vi "Measure_Synthetic_Jet_Select_Channel.vi"(3 "Mode":T1=enum."Run VI", 5 "Traverse line In":T3={"Start X"=0.0, "Start Y"=0.0, "Start Z"=0.0, "End X"=nan, "End Y"=nan, "End Z"=nan, "No. of pts."=5, "Spacing"=enum."Linear", "Filename"=path "C:/EnFlo_Data_Local/2013/Aero_Tunnel/Nick_Martin/Results/01-2013/QA_test_I.xls", "Tunnel Speed"=nan, "Averaging time (min)"=0.08, "Extra Commands"="", "Specific Arguments"="Measure_Synthetic_Jet.vi; 200; 1000; 100", "Emission Rate (l/min)"=nan, "Trace Gas Concentration (%)"=nan, "Density Ratio"="  ---------", "Comments"="", "Row No"=0, "Row Type Selector"=enum."Run VI Named:", "Completion time"="17:12  07-01-2013", "Row Duration (mins)"=4.483248000000001, "No. of Valid pts."=5, "Meas Setup File"="LDA_SJ_A.xls"} {"Row Duration (mins)" format="%#.1f"; "Row No" min=0; "Trace Gas Concentration (%)" min=0.0 format="%#.2f"; "Emission Rate (l/min)" format="%#.2f"; "Tunnel Speed" format="%#.2f"; "Start X" format="%#.2f"; "Start Y" format="%#.2f"; "Start Z" format="%#.2f"; "End X" format="%#.2f"; "End Y" format="%#.2f"; "End Z" format="%#.2f"; "Averaging time (min)" min=0.0 format="%#.2f"}) -> (0 "Error Message":string, 1 "Status":T2, 2 "Traverse line Out":T3={"Start X"=0.0, "Start Y"=0.0, "Start Z"=0.0, "End X"=nan, "End Y"=nan, "End Z"=nan, "No. of pts."=5, "Spacing"=enum."Linear", "Filename"=path "C:/EnFlo_Data_Local/2013/Aero_Tunnel/Nick_Martin/Results/01-2013/QA_test_I.xls", "Tunnel Speed"=nan, "Averaging time (min)"=0.08, "Extra Commands"="", "Specific Arguments"="Measure_Synthetic_Jet.vi; 200; 1000; 100", "Emission Rate (l/min)"=nan, "Trace Gas Concentration (%)"=nan, "Density Ratio"="  ---------", "Comments"="", "Row No"=0, "Row Type Selector"=enum."Run VI Named:", "Completion time"="17:12  07-01-2013", "Row Duration (mins)"=4.483248000000001, "No. of Valid pts."=5, "Meas Setup File"="LDA_SJ_A.xls"} {"Row Duration (mins)" format="%#.1f"; "Row No" min=0; "Trace Gas Concentration (%)" min=0.0 format="%#.2f"; "Emission Rate (l/min)" format="%#.2f"; "Tunnel Speed" format="%#.2f"; "Start X" format="%#.2f"; "Start Y" format="%#.2f"; "Start Z" format="%#.2f"; "End X" format="%#.2f"; "End Y" format="%#.2f"; "End Z" format="%#.2f"; "Averaging time (min)" min=0.0 format="%#.2f"})   [LabVIEW 2013]
uses:
  Gen Trav/Traverse_cluster.ctl
  Gen Trav/Spacing.ctl
  Controls/Multi_run_mode.ctl
  Gen Trav/Multi_Run_Status.ctl
  Controls/User_Specific_mode.ctl
  Controls/Setup.ctl
  Controls/Save_Data.ctl
  ADAM Client/Sub VIs/ADAM Controls/Update_scan_value.ctl
  <vilib>/Analysis/1siggen.llb/Ramp Pattern by Samples.vi
  Globals/Meas_global.vi
  Globals/Synthetic_jet_global.vi
  Globals/Extra_Commands_Global.vi
  <vilib>/Analysis/NI_AALBase.lvlib
panel:
  in  "Ch2 Phse average? (ON for AM on Ch2)":bool
  in  "Enter SJ Data?":bool
  in  "Stop Button":bool
  out "Last Meas Point":bool=TRUE
  out "Data":cluster{"Ramp Pattern":dbl[], dbl[]}[](graph)
  in  "Channels to Analyse":i32[](listbox)=[0, 2]
  in  "VISA resource name":refnum<visa-resource-name>="USB0::0x0699::0x0347::C036837::INSTR"
  out "First Meas Point":bool=TRUE
  # "Check the Multirun in order to populate these Channels!"
  # "X           Y            Z"
  # "Start"
  # "End"
  # "X           Y            Z"
  # "Start"
  # "End"
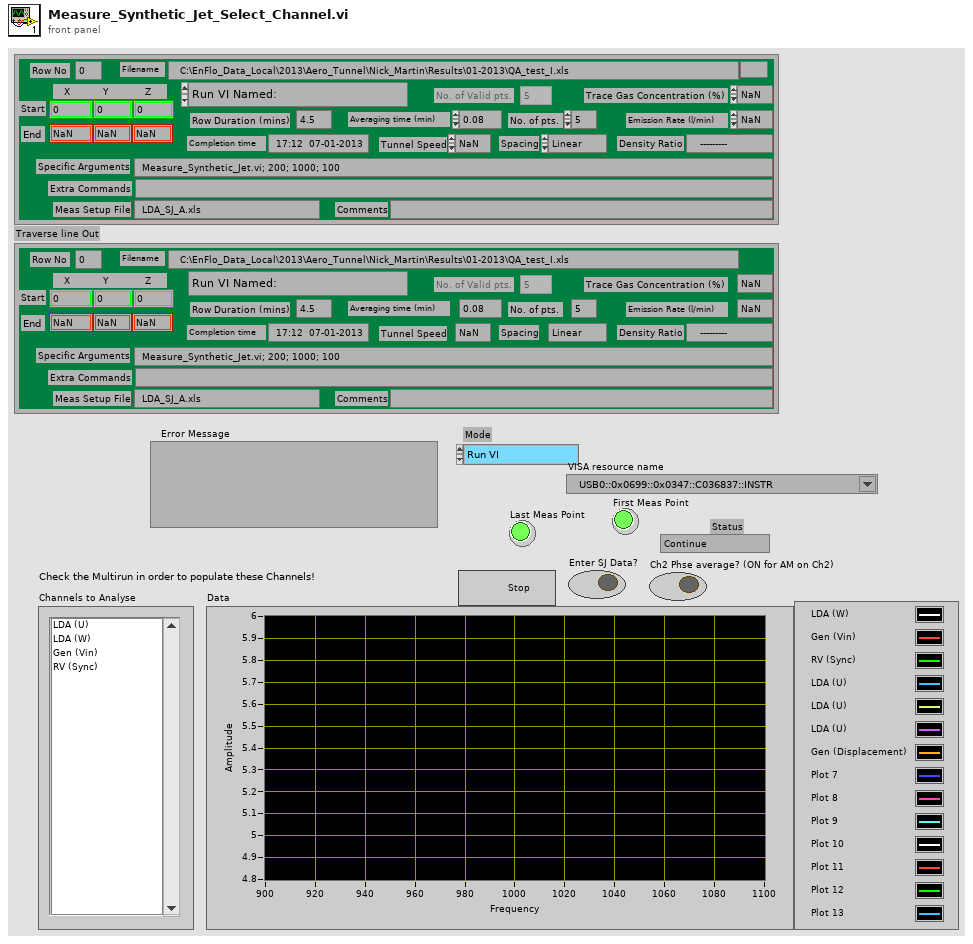
[diagram p1: front panel]
types:
  T1 = typedef "User_Specific_mode.ctl" = enum16{"Check VI only", "Run VI"}
  T2 = typedef "Multi_Run_Status.ctl" = enum16{"Continue", "Jump to Next Point", "Jump to Next Row", "Jump To Fall Back", "Terminate Run"}
  T3 = typedef "Traverse_cluster.ctl" = cluster{"Start X":dbl, "Start Y":dbl, "Start Z":dbl, "End X":dbl, "End Y":dbl, "End Z":dbl, "No. of pts.":i32, "Spacing":T4, "Filename":path, "Tunnel Speed":dbl, "Averaging time (min)":dbl, "Extra Commands":string, "Specific Arguments":string, "Emission Rate (l/min)":dbl, "Trace Gas Concentration (%)":dbl, "Density Ratio":string, "Comments":string, "Row No":i32, "Row Type Selector":T5, "Completion time":string, "Row Duration (mins)":dbl, "No. of Valid pts.":i32, "Meas Setup File":string}
  T4 = typedef "Spacing.ctl" = enum16{"Linear", "Log", "Gauss", "Specified", "N/A"}
  T5 = typedef "Multi_run_mode.ctl" = enum16{"Move Traverse Only", "Set Tunnel Speed Only", "Set Source Only", "Set Measurement Conditions", "Single Measurement", "Vertical Profile", "Lateral Profile", "Longitudinal Profile", "Explore Volume", "Multi-Axis Profile", "Auto Calibrate", "Meas Fast FID Bkgnd", "Check Beam Power", "Scanning Valve Measurement", "Run VI Named:", "Set ADAM Ch", "Wait (minutes)", "Send Message", "Synchronize With:", "Fall Back to this Row", "Turn Off Row Repeating", "Blank Row", "Traverse 3D Volume"}
  T6 = typedef "Analysis_info_cluster.ctl" = cluster{"Colour":u32, "Inst type":T7, "Inst name":string, "Symbol":string, "Code name":string, "Extra Info":string, "Inst Array":T8, "Extra Titles":string[], "Extra Values":string[], "U":dbl, "u^2":dbl, "u^3":dbl, "u^4":dbl, "Skew_u":dbl, "Kurt_u":dbl, "Sd Error in Mean":dbl, "% u'/U":dbl, "X":dbl, "Y":dbl, "Z":dbl, "Timescale integral to 25%":dbl, "Sd Error in Variance":dbl, "Calib File":path, "Calib Constants":dbl[], "Output Position":bool, "Full Stats":bool, "Av Sampling Rate":dbl, "Av No of Samples":dbl, "Total Meas Time (s)":dbl, "ADAM Ch Name":string}
  T7 = typedef "Inst_type.ctl" = enum16{"Propeller anemometer", "Raw voltage", "Pressure Transducer", "Pitot-static tube", "Preston tube", "Hot wire", "Cross wire 1", "Cross wire 2", "Generic Linear", "Generic Polynomial", "Generic BackPoly", "Fast FID", "Thermocouple", "Cold wire", "Pulsed Wire", "LDA Vel", "LDA Tran time", "LDA Arr time"}
  T8 = typedef "Instrument_Array.ctl" = enum16{"PWA", "LDA", "Analogue"}
  T9 = typedef "Save_Data.ctl" = enum16{"Save No Data", "Save Data"}
  T10 = typedef "Setup.ctl" = enum16{"Run Program", "Show Setup", "Save Current Setup", "Setup Front Panel"}
  T11 = typedef "SJ_Data_Cluster.ctl" = cluster{"Do (mm)":dbl, "Dc (mm)":dbl, "Ho (mm)":dbl, "Hc (mm)":dbl, "K":dbl, "beta":dbl, "Vc (m^3)":dbl, "Vo (m^3)":dbl}
  T12 = typedef "Update_scan_value.ctl" = cluster{"Channel Name":string, "New Value":dbl}
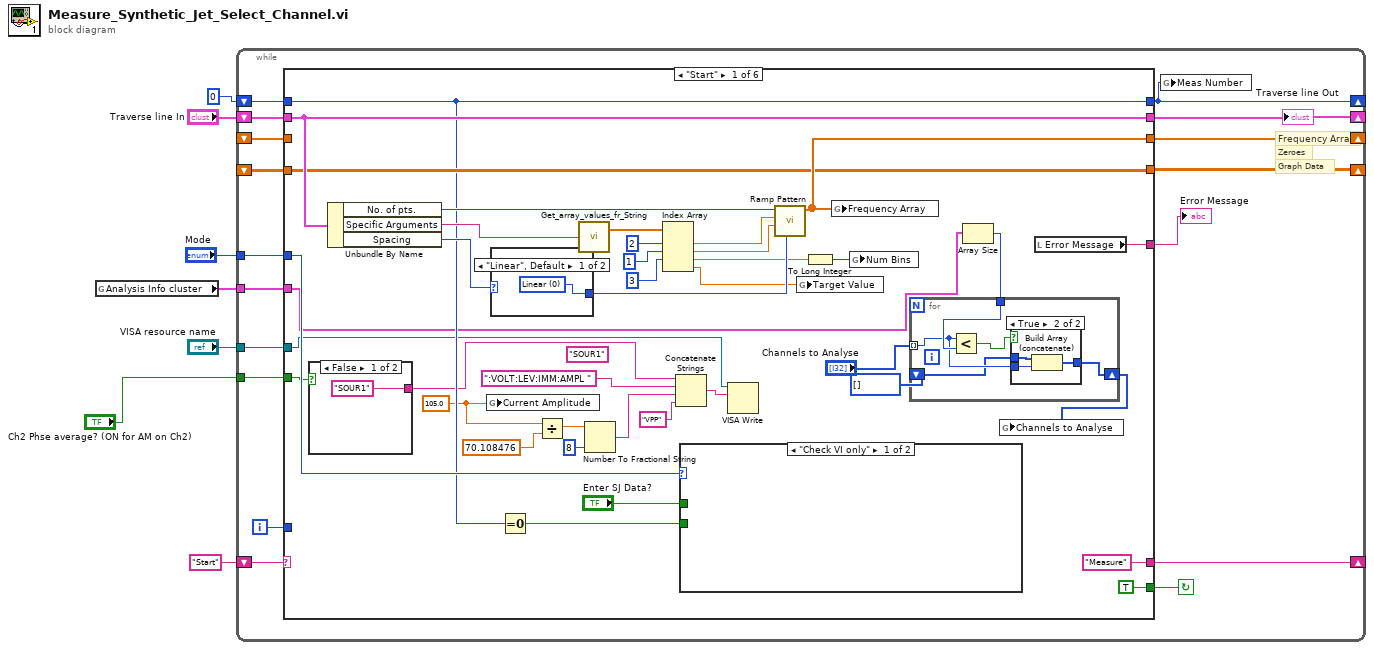
[diagram p0: block diagram]
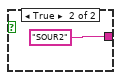
[diagram p2: hidden frame]
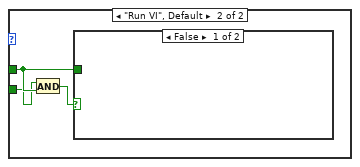
[diagram p4: hidden frame]
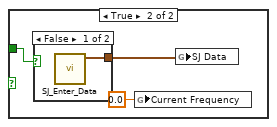
[diagram p5: hidden frame]
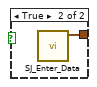
[diagram p6: hidden frame]
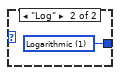
[diagram p7: hidden frame]
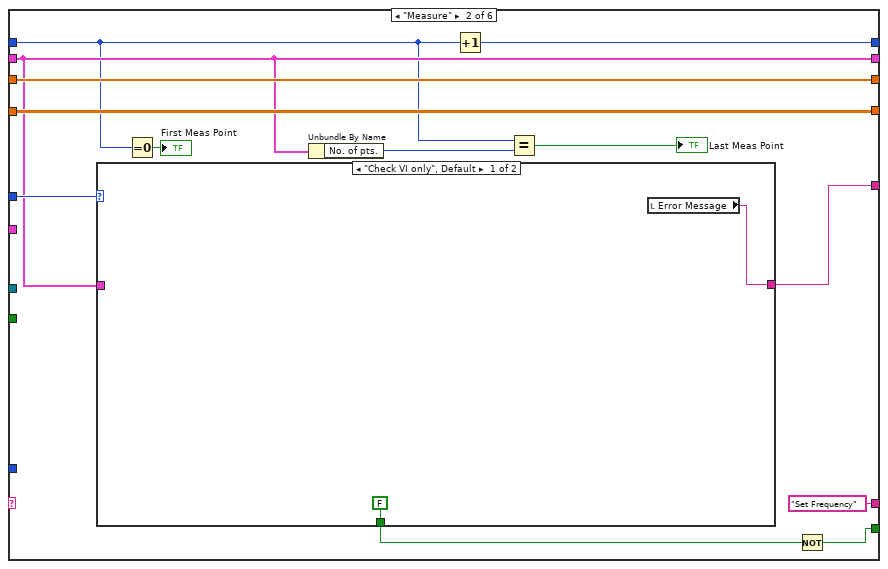
[diagram p8: hidden frame]
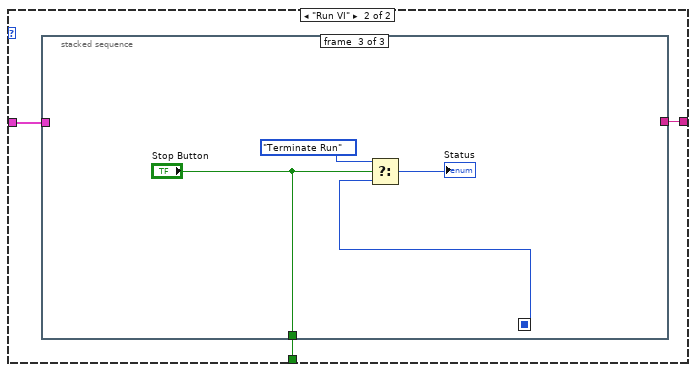
[diagram p9: hidden frame]
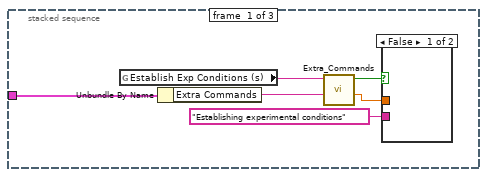
[diagram p10: hidden frame]
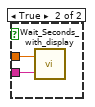
[diagram p11: hidden frame]
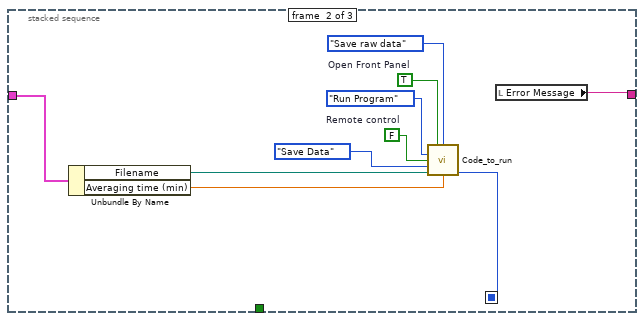
[diagram p12: hidden frame]
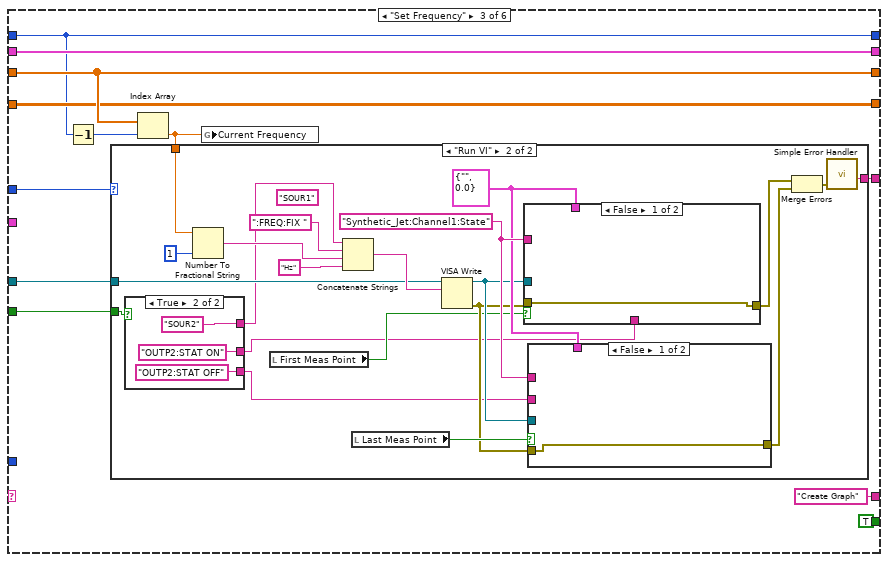
[diagram p13: hidden frame]
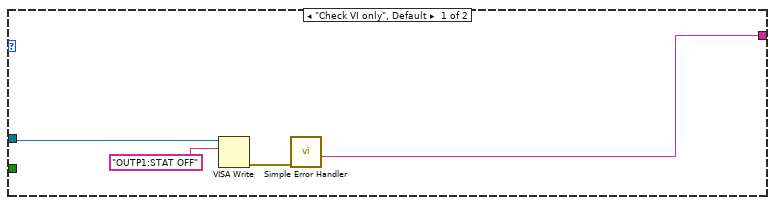
[diagram p14: hidden frame]
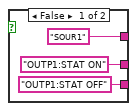
[diagram p15: hidden frame]
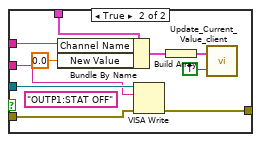
[diagram p16: hidden frame]
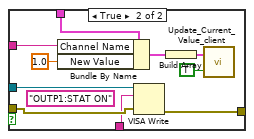
[diagram p17: hidden frame]
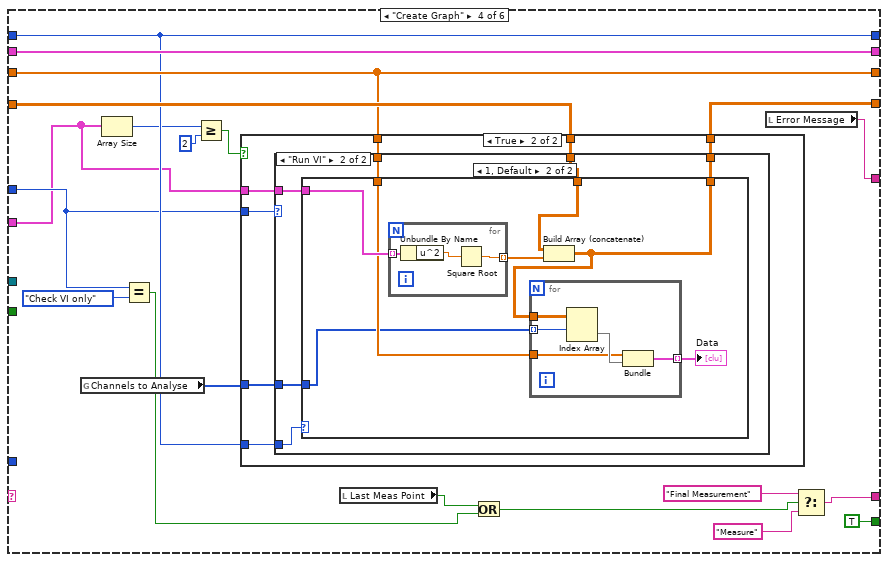
[diagram p18: hidden frame]
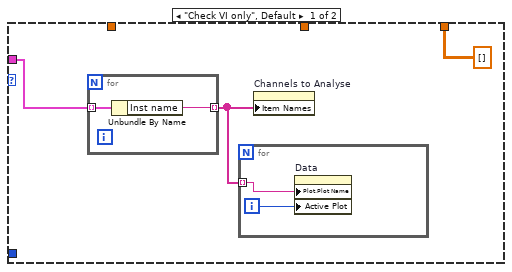
[diagram p20: hidden frame]
diagram:
  # "Graph Data"
  # "Zeroes"
  # "Frequency Array"
  n1 = global read "Meas_global.vi" "Analysis Info cluster"() -> (w2:T6[])
  n2 = while {
    shift-right: [w23] -> _
    shift-left: "Start" -> [w22]
    shift-right: [w21] -> w6
    shift-left: "Traverse line In" -> [w25]
    shift-right: [w20] -> _
    shift-left: _ -> [w19]
    tunnel: "Mode" -> [w18]
    tunnel: "VISA resource name" -> [w16]
    shift-right: [w15] -> _
    shift-left: _ -> [w14]
    shift-right: [w11] -> _
    shift-left: 0 -> [w12]
    tunnel: w2 -> [w10]
    tunnel: "Ch2 Phse average? (ON for AM on Ch2)" -> [w9]
    i -> [w17]
    stop <- w24 continue-if-true
    n3 = case shown="\"Start\"" w22 {
      selector: w22 -> [_ _ _ _ _ w265]
      tunnel: w25 -> [w62 w92 w135 w210 w258 w273]
      tunnel: [TRUE w86 TRUE TRUE ("Last Meas Point") FALSE ("Last Meas Point") FALSE] -> w24
      tunnel: ["Measure" "Set Frequency" "Create Graph" w204 "" ""] -> w23
      tunnel: [w62 w92 w135 w210 w258 w273] -> w21
      tunnel: [w50 w97 w134 w207 dbl[] [] ("Ramp Pattern") w264] -> w20
      tunnel: w19 -> [_ w97 w134 w207 _ w264]
      tunnel: w18 -> [w51 w96 w130 w200 _ _]
      tunnel: w17 -> [_ _ _ _ _ _]
      tunnel: w16 -> [w37 _ w131 _ _ _]
      tunnel: [w49 w95 w129 w209 dbl[][] [] w263] -> w15
      tunnel: w14 -> [w49 w95 w129 w208 _ w263]
      tunnel: [w48 w94 w128 w206 w257 w262] -> w13
      tunnel: [w44 w90 w127 w201 w254 w261] -> w11
      tunnel: w12 -> [w44 w88 w127 w201 w254 w261]
      tunnel: w10 -> [w32 _ _ w191 _ _]
      tunnel: w9 -> [w26 _ w126 _ _ _]
      frame "Start" {
        w34 = 105.0 ("number")
        (unwired) "SOUR1" ("string")
        n4 = case shown="False" w26 {
          tunnel: ["SOUR1" "SOUR2"] -> w27
          frame False {
          }
          frame True {
          }
        }
        n5 = Unbundle By Name(w62) -> ("No. of pts."=w61:i32, "Specific Arguments"=w58:string, "Spacing"=w60:T4)
        n6 = global write "Synthetic_jet_global.vi" "Current Amplitude"(w34) -> ()
        n7 = case shown="\"Linear\", Default" w60 {
          tunnel: [w84 w85] -> w59
          frame "Linear", Default {
            w84 = u16 0 items=["Linear", "Logarithmic"] ("type")
          }
          frame "Log" {
            w85 = u16 1 items=["Linear", "Logarithmic"] ("type")
          }
        }
        n8 = Equal To 0?(x=w44) -> (x = 0?=w52:bool)
        n9 = Divide(x=w34, y=70.108476) -> (x/y=w36:dbl)
        n10 = call "Get_array_values_fr_String.vi"("String Value"=w58) -> ("Numeric Array"=w57:dbl[])  [unwired: 1 out]
        n11 = Number To Fractional String(number=w36, precision (6)=i16 8) -> (F-format string=w39:string)  [unwired: 2 in]
        n12 = Index Array(array=w57, index #1=2 ("index"), index #2=1 ("index"), index #3=3 ("index")) -> (element #1=w54:dbl, element #2=w53:dbl, element #3=w46:dbl, element #4=w43:dbl)  [unwired: 1 in]
        n13 = Concatenate Strings(w27, ":VOLT:LEV:IMM:AMPL " ("string"), w39, "VPP" ("string")) -> (w40:string)
        n14 = case shown="\"Check VI only\"" w51 {
          tunnel: w52 -> [_ w77]
          tunnel: "Enter SJ Data?" -> [_ w78]
          frame "Check VI only" {
          }
          frame "Run VI", Default {
            n15 = And(x=w77, y=w78) -> (x .and. y?=w76:bool)
            n16 = case shown="False" w76 {
              tunnel: w78 -> [_ w80]
              frame False {
              }
              frame True {
                n17 = case shown="False" w80 {
                  tunnel: [w82 w83] -> w79
                  frame False {
                    n18 = call "SJ_Enter_Data.vi"() -> ("SJ Data"=w82:T11)  [unwired: 11 in]
                  }
                  frame True {
                    n19 = call "SJ_Enter_Data.vi"() -> ("SJ Data"=w83:T11)  [unwired: 11 in]
                  }
                }
                n20 = global write "Synthetic_jet_global.vi" "Current Frequency"(0.0 ("Current Frequency")) -> ()
                n21 = global write "Synthetic_jet_global.vi" "SJ Data"(w79) -> ()
              }
            }
          }
        }
        n22 = VISA Write(VISA resource name=w37, write buffer=w40) -> ()  [unwired: 1 in, 3 out]
        n23 = call-poly <vilib>:"Ramp Pattern.vi"("type"=w59, "start"=w53, "end"=w54, "samples"=w61) -> ("Ramp Pattern"=w50:dbl[])  [unwired: 6 in, 1 out]
        n24 = global write "Synthetic_jet_global.vi" "Target Value"(w43) -> ()
        n25 = To Long Integer(number=w46) -> (32bit integer=w45:i32)
        n26 = global write "Synthetic_jet_global.vi" "Frequency Array"(w50) -> ()
        n27 = global write "Synthetic_jet_global.vi" "Num Bins"(w45) -> ()
        n28 = Array Size(array=w32) -> (size(s)=w33:i32)
        n29 = for {
          tunnel: w33 -> [w71]
          tunnel: "Channels to Analyse" -> [w69] mode=indexing
          shift-right: [w68] -> w30
          shift-left: i32[] [] -> [w67]
          n30 = Less?(x=w69, y=w71) -> (x < y?=w70:bool)
          n31 = case shown="True" w70 {
            tunnel: w69 -> [_ w75]
            tunnel: [w72 w74] -> w68
            tunnel: w67 -> [w72 w73]
            frame False {
            }
            frame True {
              n32 = Build Array (concatenate)(w73, w75) -> (w74:i32[])
            }
          }
        }
        n33 = global write "Synthetic_jet_global.vi" "Channels to Analyse"(w30) -> ()
        n34 = local read "Error Message"() -> (w48:string)
      }
      frame "Measure" {
        n35 = case shown="\"Check VI only\", Default" w96 {
          tunnel: w92 -> [_ w103]
          tunnel: [w100 w102] -> w94
          tunnel: [FALSE ("Stop Button") w101] -> w87
          frame "Check VI only", Default {
            n36 = local read "Error Message"() -> (w100:string)
          }
          frame "Run VI" {
            n37 = stacked-sequence {
              seq-local: [_ w112 _] -> [_ _ w123]
              tunnel: w103 -> [w104 w117 _]
              tunnel: [_ w114 _] -> w102
              tunnel: [_ _ "Stop Button"] -> w101
              frame #0 {
                n38 = global read "Extra_Commands_Global.vi" "Establish Exp Conditions (s)"() -> (w107:string)
                n39 = Unbundle By Name(w104) -> ("Extra Commands"=w105:string)
                n40 = call "Extra_Commands.vi"("String to Search"=w105, "Command"=w107) -> ("Numeric Value"=w106:dbl, "Command Found"=w108:bool)  [unwired: 2 in, 2 out]
                n41 = case shown="False" w108 {
                  tunnel: w106 -> [_ w111]
                  tunnel: "Establishing experimental conditions" ("Message") -> [_ w110]
                  frame False {
                  }
                  frame True {
                    n42 = call "Wait_Seconds_with_display.vi"("Message"=w110, "Seconds to wait"=w111) -> ()  [unwired: 1 in, 1 out]
                  }
                }
              }
              frame #1 {
                w119 = TRUE  # Open Front Panel
                w118 = FALSE  # Remote control
                n43 = Unbundle By Name(w117) -> ("Filename"=w116:path, "Averaging time (min)"=w113:dbl)
                n44 = call "Code_to_run.vi"("Open Front Panel"=w119, "Raw data option"=enum16{"Save raw data", "Raw data not saved"}."Save raw data", "setup"=Setup."Run Program", "Remote control"=w118, "File"=Save_Data."Save Data", "Results Filename"=w116, "Averaging time (min)"=w113) -> ("Status"=w112:T2)  [unwired: 4 in, 4 out]
                n45 = local read "Error Message"() -> (w114:string)
              }
              frame #2 {
                n46 = Select(t=Multi_Run_Status."Terminate Run", s="Stop Button", f=w123) -> (s? t:f=→"Status":T2)
              }
            }
          }
        }
        n47 = Equal To 0?(x=w88) -> (x = 0?=→"First Meas Point":bool)
        n48 = Unbundle By Name(w92) -> ("No. of pts."=w91:i32)
        n49 = Increment(x=w88) -> (x+1=w90:i32)
        n50 = Equal?(x=w88, y=w91) -> (x = y?=→"Last Meas Point":bool)
        n51 = Not(x=w87) -> (.not. x?=w86:bool)
      }
      frame "Set Frequency" {
        n52 = Decrement(x=w127) -> (x-1=w133:i32)
        n53 = Index Array(array=w134, index=w133) -> (element=w132:dbl)
        n54 = case shown="\"Run VI\"" w130 {
          tunnel: w132 -> [_ w155]
          tunnel: w131 -> [w140 w154]
          tunnel: [w138 w151] -> w128
          tunnel: w126 -> [_ w142]
          frame "Check VI only", Default {
            n55 = VISA Write(VISA resource name=w140, write buffer="OUTP1:STAT OFF") -> (error out=w139:errorcluster)  [unwired: 1 in, 2 out]
            n56 = call <vilib>:"Simple Error Handler.vi"("error in (no error)"=w139) -> ("source out"=w138:string)  [unwired: 4 in, 4 out]
          }
          frame "Run VI" {
            w156 = T12 {"Channel Name"="", "New Value"=0.0} ("Update Scan Value Cluster")
            w157 = "Synthetic_Jet:Channel1:State" ("write buffer")
            (unwired) "SOUR1"
            n57 = case shown="True" w142 {
              tunnel: ["SOUR1" "SOUR2"] -> w145
              tunnel: ["OUTP1:STAT ON" ("write buffer") "OUTP2:STAT ON" ("write buffer")] -> w144
              tunnel: ["OUTP1:STAT OFF" ("write buffer") "OUTP2:STAT OFF" ("write buffer")] -> w143
              frame False {
              }
              frame True {
              }
            }
            n58 = Number To Fractional String(number=w155, precision (6)=i16 1) -> (F-format string=w160:string)  [unwired: 2 in]
            n59 = local read "First Meas Point"() -> (w146:bool)
            n60 = Concatenate Strings(w145, ":FREQ:FIX " ("string"), w160, "Hz" ("string")) -> (w162:string)
            n61 = local read "Last Meas Point"() -> (w153:bool)
            n62 = VISA Write(VISA resource name=w154, write buffer=w162) -> (VISA resource name out=w152:refnum<visa-resource-name>, error out=w147:errorcluster)  [unwired: 1 in, 1 out]
            n63 = case shown="False" w146 {
              tunnel: w157 -> [_ w186]
              tunnel: w156 -> [_ w185]
              tunnel: w152 -> [_ w184]
              tunnel: [w180 w183] -> w148
              tunnel: w147 -> [w180 w182]
              tunnel: w144 -> [_ w181]
              frame False {
              }
              frame True {
                (unwired) "OUTP1:STAT ON" ("write buffer")
                n64 = Bundle By Name(cluster=w185, "Channel Name"=w186, "New Value"=1.0) -> (w189:T12)
                n65 = VISA Write(VISA resource name=w184, write buffer=w181, error in (no error)=w182) -> (error out=w183:errorcluster)  [unwired: 2 out]
                n66 = Build Array(w189) -> (w188:T12[])
                n67 = call "Update_Current_Value_client.vi"("Don't Bother with check?"=TRUE, "Update array in"=w188) -> ()
              }
            }
            n68 = case shown="False" w153 {
              tunnel: w157 -> [_ w175]
              tunnel: w156 -> [_ w174]
              tunnel: w152 -> [_ w173]
              tunnel: [w169 w172] -> w149
              tunnel: w147 -> [w169 w171]
              tunnel: w143 -> [_ w170]
              frame False {
              }
              frame True {
                (unwired) "OUTP1:STAT OFF" ("write buffer")
                n69 = Bundle By Name(cluster=w174, "Channel Name"=w175, "New Value"=0.0) -> (w178:T12)
                n70 = VISA Write(VISA resource name=w173, write buffer=w170, error in (no error)=w171) -> (error out=w172:errorcluster)  [unwired: 2 out]
                n71 = Build Array(w178) -> (w177:T12[])
                n72 = call "Update_Current_Value_client.vi"("Don't Bother with check?"=TRUE, "Update array in"=w177) -> ()
              }
            }
            n73 = Merge Errors(w148, w149) -> (w150:errorcluster)
            n74 = call <vilib>:"Simple Error Handler.vi"("error in (no error)"=w150) -> ("source out"=w151:string)  [unwired: 4 in, 4 out]
          }
        }
        n75 = global write "Synthetic_jet_global.vi" "Current Frequency"(w132) -> ()
      }
      frame "Create Graph" {
        n76 = global read "Synthetic_jet_global.vi" "Channels to Analyse"() -> (w192:i32[])
        n77 = Array Size(array=w191) -> (size(s)=w193:i32)
        n78 = Equal?(x=w200, y=User_Specific_mode."Check VI only") -> (x = y?=w197:bool)
        n79 = Greater Or Equal?(x=w193, y=2 ("x")) -> (x >= y?=w195:bool)
        n80 = case shown="True" w195 {
          tunnel: w191 -> [_ w218]
          tunnel: [w211 w217] -> w209
          tunnel: w208 -> [w211 w216]
          tunnel: w207 -> [_ w215]
          tunnel: w201 -> [_ w214]
          tunnel: w200 -> [_ w213]
          tunnel: w192 -> [_ w212]
          frame False {
          }
          frame True {
            n81 = case shown="\"Run VI\"" w213 {
              tunnel: w218 -> [w221 w231]
              tunnel: w214 -> [_ w230]
              tunnel: [dbl[][] [] w229] -> w217
              tunnel: w216 -> [_ w228]
              tunnel: w215 -> [_ w227]
              tunnel: w212 -> [_ w226]
              frame "Check VI only", Default {
                n82 = for {
                  tunnel: w221 -> [w225] mode=indexing
                  tunnel: [w224] -> w219 mode=indexing
                  n83 = Unbundle By Name(w225) -> ("Inst name"=w224:string)
                }
                n84 = for {
                  tunnel: w219 -> [w223] mode=indexing
                  i -> [w222]
                  n85 = property on="Data" class="XYGraph (strict)"("Plot.Plot Name"=w223, "Active Plot"=w222) -> ()  [unwired: 2 in, 2 out]
                }
                n86 = property on="Channels to Analyse" class="LstBox (strict)"("Item Names"=w219) -> ()  [unwired: 2 in, 2 out]
              }
              frame "Run VI" {
                n87 = case shown="1, Default" w230 {
                  tunnel: w231 -> [w234 w245]
                  tunnel: [dbl[][] [] w242] -> w229
                  tunnel: w228 -> [_ w243]
                  tunnel: w227 -> [_ w241]
                  tunnel: w226 -> [_ w239]
                  frame 0 {
                    n88 = for {
                      tunnel: w234 -> [w238] mode=indexing
                      tunnel: [w237] -> w232 mode=indexing
                      n89 = Unbundle By Name(w238) -> ("Inst name"=w237:string)
                    }
                    n90 = for {
                      tunnel: w232 -> [w236] mode=indexing
                      i -> [w235]
                      n91 = property on="Data" class="XYGraph (strict)"("Plot.Plot Name"=w236, "Active Plot"=w235) -> ()  [unwired: 2 in, 2 out]
                    }
                    n92 = property on="Channels to Analyse" class="LstBox (strict)"("Item Names"=w232) -> ()  [unwired: 2 in, 2 out]
                  }
                  frame 1, Default {
                    n93 = for {
                      tunnel: w245 -> [w253] mode=indexing
                      tunnel: [w251] -> w244 mode=indexing
                      n94 = Unbundle By Name(w253) -> ("u^2"=w252:dbl)
                      n95 = Square Root(x=w252) -> (sqrt(x)=w251:dbl)
                    }
                    n96 = Build Array (concatenate)(w243, w244) -> (w242:dbl[][])
                    n97 = for {
                      tunnel: w242 -> [w250]
                      tunnel: w239 -> [w246] mode=indexing
                      tunnel: w241 -> [w248]
                      tunnel: [w247] -> w240 mode=indexing
                      n98 = Index Array(array=w250, index (row)=w246) -> (element=w249:dbl[])  [unwired: 1 in]
                      n99 = Bundle("Ramp Pattern"=w248, w249) -> (w247:cluster{"Ramp Pattern":dbl[], dbl[]})  [unwired: 1 in]
                    }
                    "Data" <- w240
                  }
                }
              }
            }
          }
        }
        n100 = local read "Last Meas Point"() -> (w198:bool)
        n101 = Or(x=w198, y=w197) -> (x .or. y?=w196:bool)
        n102 = local read "Error Message"() -> (w206:string)
        n103 = Select(t="Final Measurement", s=w196, f="Measure") -> (s? t:f=w204:string)
      }
      frame "Final Measurement" {
        n104 = local read "Error Message"() -> (w257:string)
      }
      frame "No Match", Default {
        n105 = Current VI's Path() -> (path=w270:path)
        n106 = Format Into String(format string="The Case\"%s\" was not Matched\nin VI named\n'%s\"" ("Format String"), w265, w270) -> (resulting string=w267:string)  [unwired: 2 in, 1 out]
        n107 = One Button Dialog(message=w267, button name ("OK")="STOP") -> (true=w269:bool)
        n108 = Stop(stop? (T)=w269) -> ()
        n109 = local read "Error Message"() -> (w262:string)
      }
    }
    "Error Message" <- w13
    n110 = global write "Synthetic_jet_global.vi" "Meas Number"(w11) -> ()
  }
  "Traverse line Out" <- w6
